vi "Update State.vi"(8 "error in (no error)":errorcluster, 10 "current_limits":dbl[](array[numeric]) min=0.0 max=0.9 step=0.01, 11 "MF3 in":refnum<class "MF3.lvclass">) -> (0 "error out":errorcluster, 3 "MF3 out":refnum<class "MF3.lvclass">)   [LabVIEW 2013, in "MF3.lvclass"]
uses:
  MF3.lvclass
  MF3.lvclass/MF3.ctl
  controls/Motor Names.ctl
  <vilib>/Utility/error.llb/Error Cluster From Error Code.vi
  <vilib>/rvi/errors/niLvFpgaAdjustHostInterfaceError.vi
  <vilib>/rvi/interface/nirviReadWriteControl/nirviReadWriteControl.xnode
  FPGA/MotorsInterface.lvbitx
  NiFpgaLv.dll
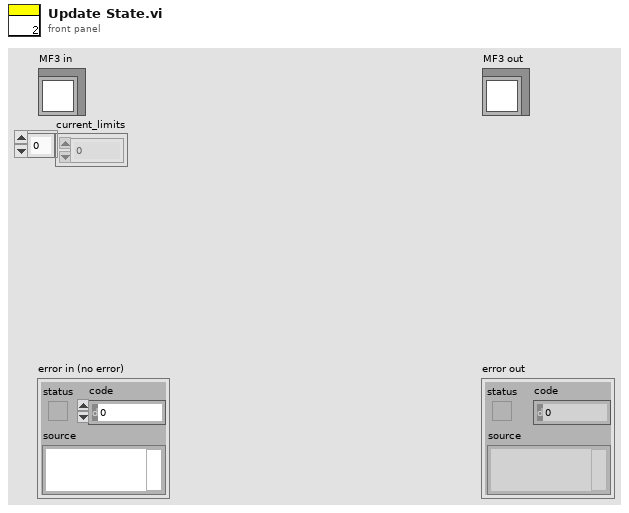
[diagram p1: front panel]
types:
  T1 = typedef "Motor Names.ctl" = enum16{"Thumb1", "Thumb2", "Thumb3", "Middle1", "Middle2", "Middle3", "Redundant", "Index1", "Index2", "Index3"}
  T2 = cluster{"Proportional Gain":i16, "Integral Gain":i16, "Derivative Gain":i16}
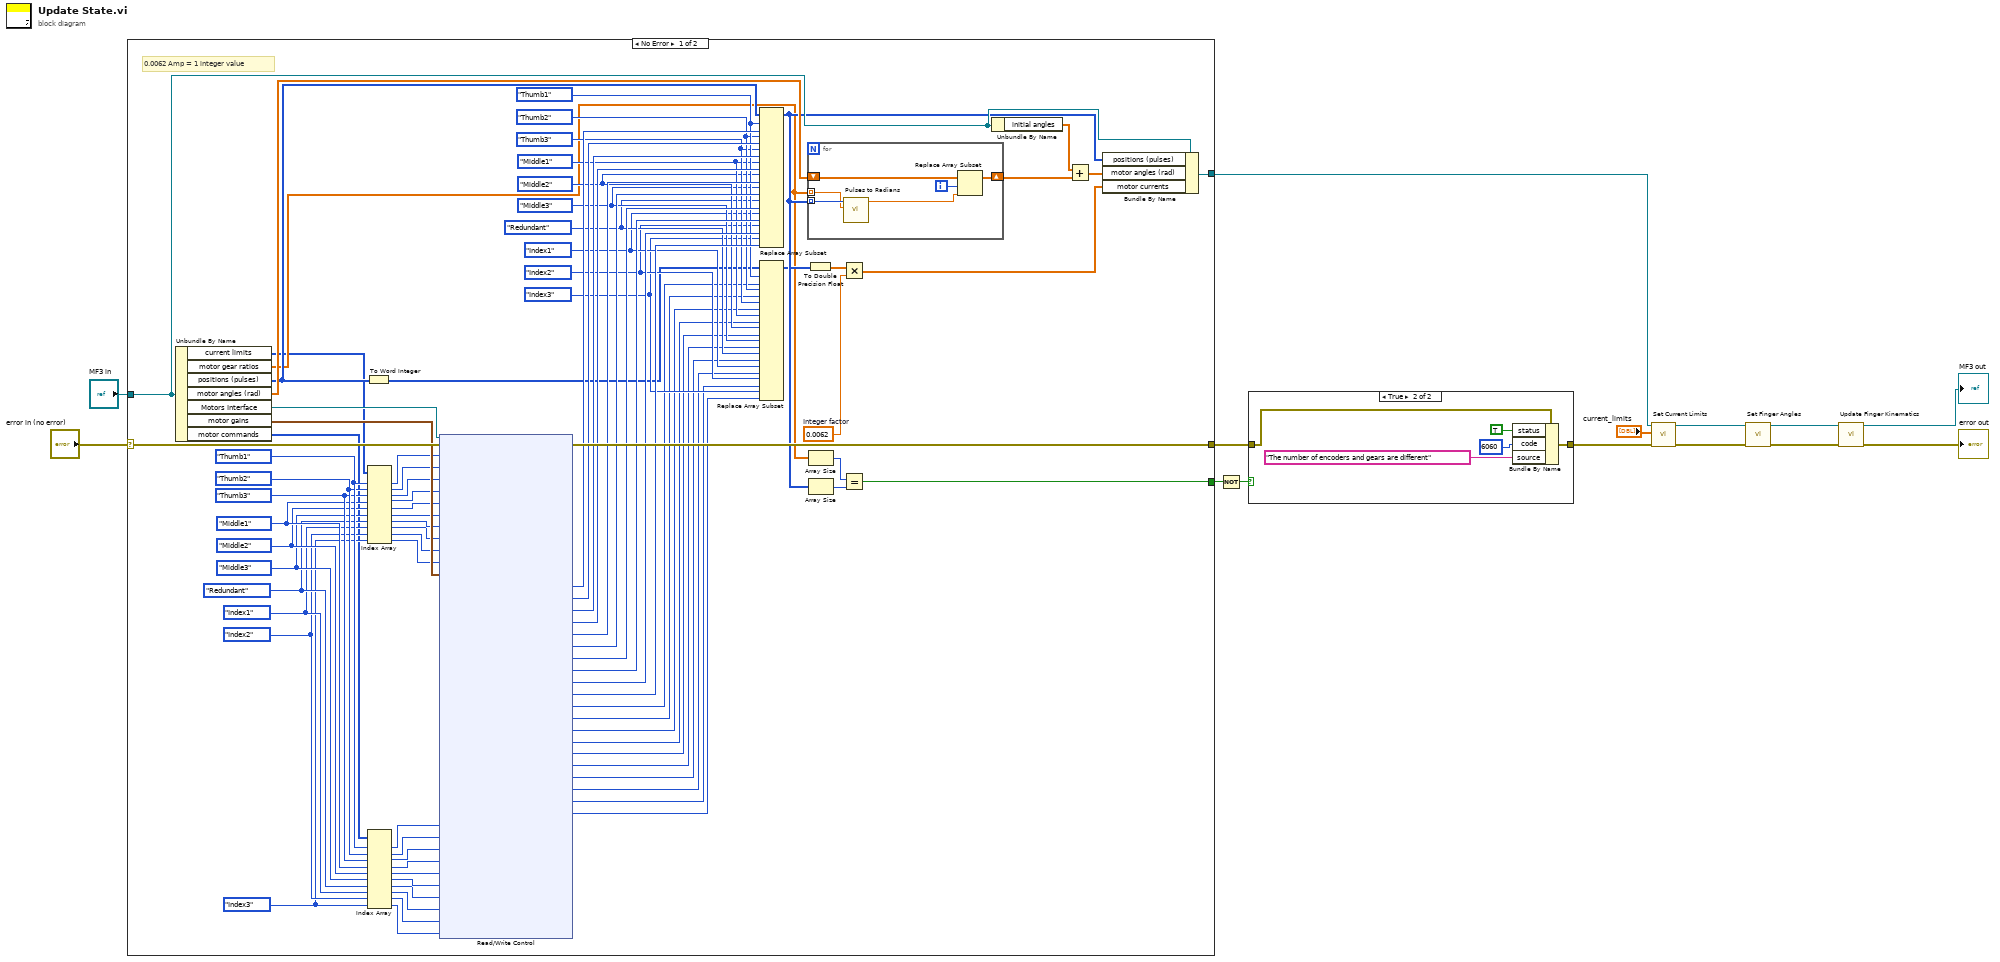
[diagram p0: block diagram]
diagram:
  n1 = case shown="No Error" "error in (no error)" {
    selector: "error in (no error)" -> [w96 w105]
    tunnel: [w95 w105] -> w8
    tunnel: [w94 w104] -> w12
    tunnel: "MF3 in" -> [w90 w104]
    tunnel: [w93 _] -> w6
    frame No Error {
      w35 = Motor_Names."Thumb1" ("Motor Names")
      w26 = Motor_Names."Index3" ("Motor Names")
      w27 = Motor_Names."Index2" ("Motor Names")
      w28 = Motor_Names."Index1" ("Motor Names")
      w29 = Motor_Names."Redundant" ("Motor Names")
      w30 = Motor_Names."Middle3" ("Motor Names")
      w31 = Motor_Names."Middle2" ("Motor Names")
      w32 = Motor_Names."Middle1" ("Motor Names")
      w33 = Motor_Names."Thumb3" ("Motor Names")
      w34 = Motor_Names."Thumb2" ("Motor Names")
      w48 = 0.0062  # Integer factor
      w67 = Motor_Names."Index3" ("Motor Names")
      w68 = Motor_Names."Index2" ("Motor Names")
      w69 = Motor_Names."Index1" ("Motor Names")
      w70 = Motor_Names."Redundant" ("Motor Names")
      w71 = Motor_Names."Middle3" ("Motor Names")
      w72 = Motor_Names."Middle2" ("Motor Names")
      w73 = Motor_Names."Middle1" ("Motor Names")
      w74 = Motor_Names."Thumb3" ("Motor Names")
      w75 = Motor_Names."Thumb2" ("Motor Names")
      w76 = Motor_Names."Thumb1" ("Motor Names")
      # "0.0062 Amp = 1 integer value"
      n2 = Unbundle By Name(w90) -> ("current limits"=w46:i16[], "motor gear ratios"=w51:dbl[], "positions (pulses)"=w63:i32[], "motor angles (rad)"=w92:dbl[], "Motors Interface"=w97:refnum<k20>, "motor gains"=w47:T2, "motor commands"=w25:i16[])
      n3 = To Word Integer(number=w63) -> (16bit integer=w62:i16[])
      n4 = Index Array(array=w46, index #1=w35, index #2=w34, index #3=w33, index #4=w32, index #5=w31, index #6=w30, index #7=w29, index #8=w28, index #9=w27, index #10=w26) -> (element #1=w45:i16, element #2=w43:i16, element #3=w42:i16, element #4=w41:i16, element #5=w40:i16, element #6=w39:i16, element #7=w38:i16, element #8=w37:i16, element #9=w36:i16, element #10=w44:i16)
      n5 = Index Array(array=w25, index #1=w35, index #2=w34, index #3=w33, index #4=w32, index #5=w31, index #6=w30, index #7=w29, index #8=w28, index #9=w27, index #10=w26) -> (element #1=w24:i16, element #2=w23:i16, element #3=w22:i16, element #4=w21:i16, element #5=w20:i16, element #6=w19:i16, element #7=w18:i16, element #8=w17:i16, element #9=w16:i16, element #10=w15:i16)
      n6 = xnode "Read/Write Control"("FPGA VI Reference In"=w97, "error in"=w96, "Current Limit Thumb 1"=w45, "Current Limit Thumb 2"=w43, "Current Limit Thumb 3"=w42, "Current Limit Middle 1"=w41, "Current Limit Middle 2"=w40, "Current Limit Middle 3"=w39, "Current Limit Redundant"=w38, "Current Limit Index 1"=w37, "Current Limit Index 2"=w36, "Current Limit Index 3"=w44, "Motors Gains"=w47, "Current Setpoint Thumb 1"=w24, "Current Setpoint Thumb 2"=w23, "Current Setpoint Thumb 3"=w22, "Current Setpoint Middle 1"=w21, "Current Setpoint Middle 2"=w20, "Current Setpoint Middle 3"=w19, "Current Setpoint Redundant"=w18, "Current Setpoint Index 1"=w17, "Current Setpoint Index 2"=w16, "Current Setpoint Index 3"=w15) -> ("error out"=w95:errorcluster, "Position Thumb 1"=w86:i32, "Position Thumb 2"=w85:i32, "Position Thumb 3"=w84:i32, "Position Middle 1"=w83:i32, "Position Middle 2"=w82:i32, "Position Middle 3"=w81:i32, "Position Redundant"=w80:i32, "Position Index 1"=w79:i32, "Position Index 2"=w78:i32, "Position Index 3"=w77:i32, "Current Thumb 1"=w64:i16, "Current Thumb 2"=w61:i16, "Current Thumb 3"=w60:i16, "Current Middle 1"=w59:i16, "Current Middle 2"=w58:i16, "Current Middle 3"=w57:i16, "Current Redundant"=w56:i16, "Current Index 1"=w55:i16, "Current Index 2"=w54:i16, "Current Index 3"=w53:i16)  [unwired: 1 out]
      n7 = Replace Array Subset(array=w63, new element #1=w86, index #1=w76, new element #2=w85, index #2=w75, new element #3=w84, index #3=w74, new element #4=w83, index #4=w73, new element #5=w82, index #5=w72, new element #6=w81, index #6=w71, new element #7=w80, index #7=w70, new element #8=w79, index #8=w69, new element #9=w78, index #9=w68, new element #10=w77, index #10=w67) -> (w66:i32[])
      n8 = Replace Array Subset(array=w62, new element #1=w64, index #1=w76, new element #2=w61, index #2=w75, new element #3=w60, index #3=w74, new element #4=w59, index #4=w73, new element #5=w58, index #5=w72, new element #6=w57, index #6=w71, new element #7=w56, index #7=w70, new element #8=w55, index #8=w69, new element #9=w54, index #9=w68, new element #10=w53, index #10=w67) -> (w65:i16[])
      n9 = for {
        shift-right: [w100] -> w91
        shift-left: w92 -> [w103]
        tunnel: w66 -> [w99] mode=indexing
        tunnel: w51 -> [w98] mode=indexing
        i -> [w102]
        n10 = call "Pulses to Radians.vi"("gear ratio"=w98, "encoder pulses"=w99) -> ("angle (rad)"=w101:dbl)  [unwired: 9 in]
        n11 = Replace Array Subset(array=w103, new element=w101, index=w102) -> (w100:dbl[])
      }
      n12 = To Double Precision Float(number=w65) -> (double precision float=w52:dbl[])
      n13 = Array Size(array=w51) -> (size(s)=w88:i32)
      n14 = Array Size(array=w66) -> (size(s)=w87:i32)
      n15 = Multiply(x=w52, y=w48) -> (x*y=w49:dbl[])
      n16 = Equal?(x=w88, y=w87) -> (x = y?=w93:bool)
      n17 = Unbundle By Name(w90) -> ("initial angles"=w89:dbl[])
      n18 = Add(x=w89, y=w91) -> (x+y=w50:dbl[])
      n19 = Bundle By Name(cluster=w90, "positions (pulses)"=w66, "motor angles (rad)"=w50, "motor currents"=w49) -> (w94:refnum<class "MF3.lvclass">)
    }
    frame Error {
    }
  }
  n20 = Not(x=w6) -> (.not. x?=w5:bool)
  n21 = case shown="True" w5 {
    tunnel: w8 -> [w106 w111]
    tunnel: [w106 w110] -> w7
    frame False {
    }
    frame True {
      n22 = Bundle By Name(cluster=w111, "status"=TRUE, "code"=6060, "source"="The number of encoders and gears are different") -> (w110:errorcluster)
    }
  }
  n23 = call "Set Current Limits.vi"("error in (no error)"=w7, "current_limits"="current_limits", "MF3 in"=w12) -> ("error out"=w10:errorcluster, "MF3 out"=w11:refnum<class "MF3.lvclass">)  [unwired: 7 in]
  n24 = call "Set Finger Angles.vi"("error in (no error)"=w10, "MF3 in"=w11) -> ("error out"=w3:errorcluster, "MF3 out"=w4:refnum<class "MF3.lvclass">)  [unwired: 8 in]
  n25 = call "Update Finger Kinematics.vi"("error in (no error)"=w3, "MF3 in"=w4) -> ("error out"=→"error out":errorcluster, "MF3 out"=→"MF3 out":refnum<class "MF3.lvclass">)  [unwired: 8 in]
